vi "虚拟放射源数据USB读取.vi"() -> ()   [LabVIEW 2013]
panel:
  out "虚拟放射源VISA":string
  in  "停止":bool
  out "数组":i32[](array[numeric])
  out "波形图":i32[](graph)
  out "随机数":u16
  in  "数据输出":u16(ring) items=["USB", "DAC"]
  in  "仪器使能":bool
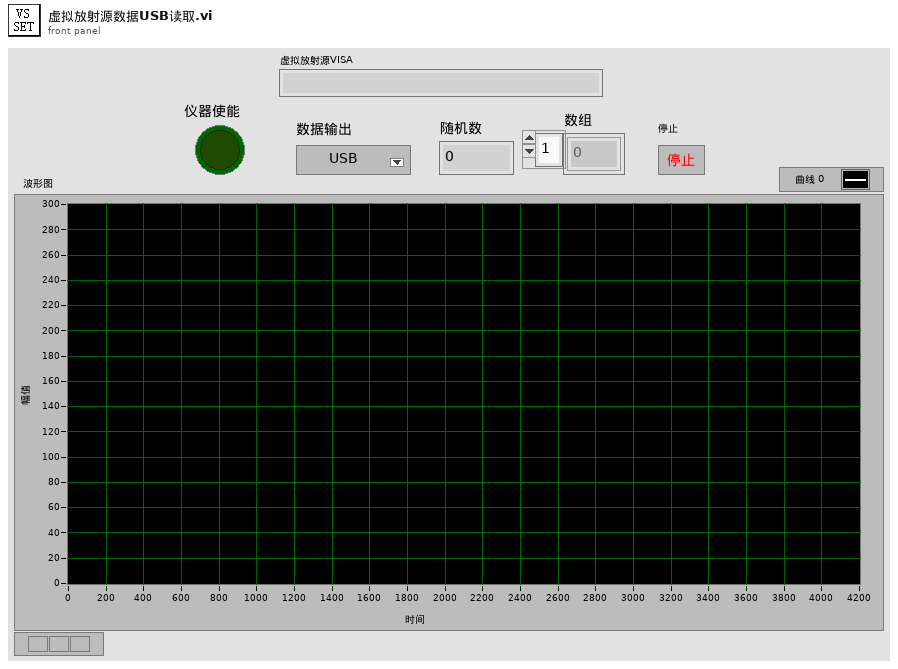
[diagram p1: front panel]
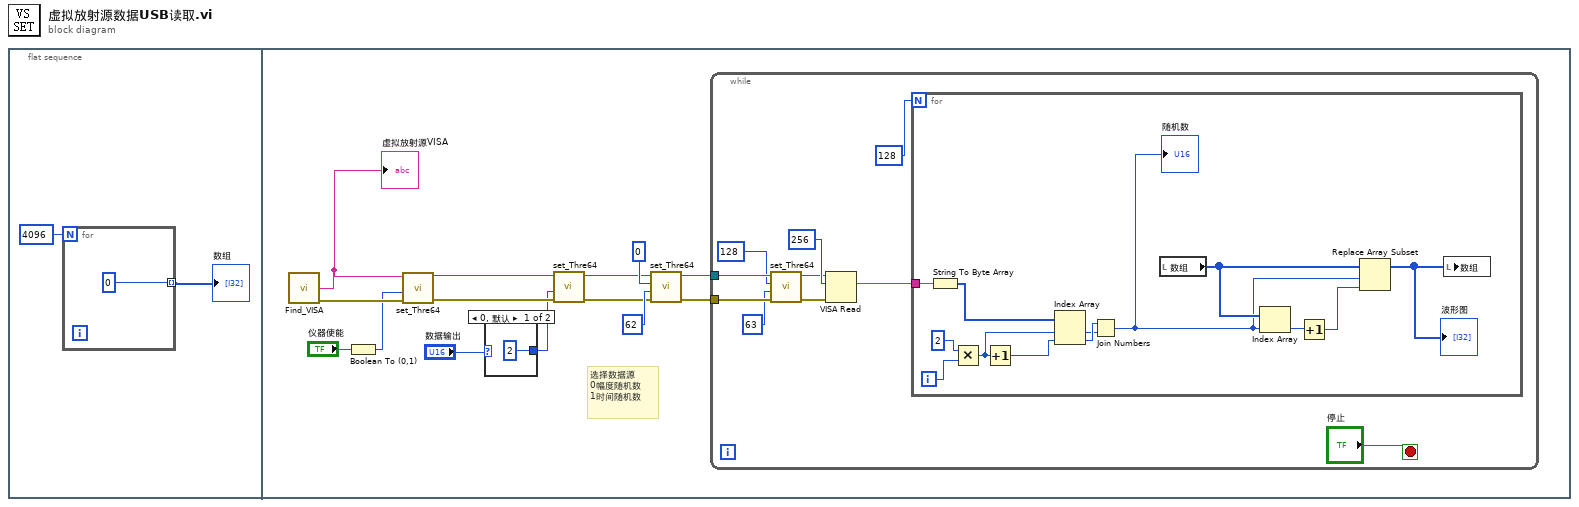
[diagram p0: block diagram]
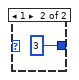
[diagram p2: hidden frame]
diagram:
  n1 = flat-sequence {
    frame #0 {
      n2 = for {
        N: 4096 -> [_]
        tunnel: [0] -> w1 mode=indexing
      }
      "数组" <- w1
    }
    frame #1 {
      # "选择数据源\n0幅度随机数\n1时间随机数"
      n3 = call "Find_VISA.vi"() -> ("错误输出"=w17:errorcluster, "虚拟放射源VISA"=w16:string)  [unwired: 3 in, 1 out]
      "虚拟放射源VISA" <- w16
      n4 = Boolean To (0,1)(Boolean="仪器使能") -> (0, 1=w14:i16)
      n5 = call "set_Thre64.vi"("错误输入（无错误）"=w17, "命令"=w14, "VISA资源名称"=w16) -> ("错误输出"=w12:errorcluster, "VISA资源名称输出"=w13:refnum<visa-resource-name>)  [unwired: 7 in]
      n6 = case shown="0, 默认" "数据输出" {
        tunnel: [2 3] -> w10
        frame 0, Default {
        }
        frame 1 {
        }
      }
      n7 = call "set_Thre64.vi"("错误输入（无错误）"=w12, "命令"=w10, "VISA资源名称"=w13) -> ("错误输出"=w6:errorcluster, "VISA资源名称输出"=w7:refnum<visa-resource-name>)  [unwired: 7 in]
      n8 = call "set_Thre64.vi"("错误输入（无错误）"=w6, "命令"=u8 62, "数字"=u16 0, "VISA资源名称"=w7) -> ("错误输出"=w4:errorcluster, "VISA资源名称输出"=w5:refnum<visa-resource-name>)  [unwired: 6 in]
      n9 = while {
        tunnel: w5 -> [w27]
        tunnel: w4 -> [w26]
        stop <- "停止" stop-if-true
        n10 = call "set_Thre64.vi"("错误输入（无错误）"=w26, "命令"=u8 63, "数字"=u16 128, "VISA资源名称"=w27) -> ("错误输出"=w22:errorcluster, "VISA资源名称输出"=w21:refnum<visa-resource-name>)  [unwired: 6 in]
        n11 = VISA Read(VISA resource name=w21, byte count=u32 256 ("字节总数"), error in (no error)=w22) -> (read buffer=w19:string)  [unwired: 3 out]
        n12 = for {
          N: 128 -> [_]
          tunnel: w19 -> [w39]
          i -> [w33]
          n13 = String To Byte Array(string=w39) -> (unsigned byte array=w36:u8[])
          n14 = Multiply(x=2, y=w33) -> (x*y=w35:i32)
          n15 = Increment(x=w35) -> (x+1=w34:i32)
          n16 = Index Array(array=w36, index #1=w35, index #2=w34) -> (element #1=w37:u8, element #2=w38:u8)
          n17 = Join Numbers(hi=w38, lo=w37) -> ((hi.lo)=w29:u16)
          "随机数" <- w29
          n18 = local read "数组"() -> (w31:i32[])
          n19 = Index Array(array=w31, index=w29) -> (element=w32:i32)
          n20 = Increment(x=w32) -> (x+1=w30:i32)
          n21 = Replace Array Subset(array=w31, new element=w30, index=w29) -> (w28:i32[])
          "波形图" <- w28
          n22 = local write "数组"(w28) -> ()
        }
      }
    }
  }
